vi "Create.vi"(8 "error in (no error)":errorcluster) -> (0 "error out":errorcluster, 3 "Mock Result Observer out":refnum<class "Mock Result Observer.lvclass">)   [LabVIEW 2020, in "Mock Result Observer.lvclass"]
uses:
  Mock Result Observer.lvclass
  Result/Result.ctl
  Result/Status.ctl
  Result/Type.ctl
  Mock Result Observer.lvclass/Mock Result Observer.ctl
  Result/Result.lvlib
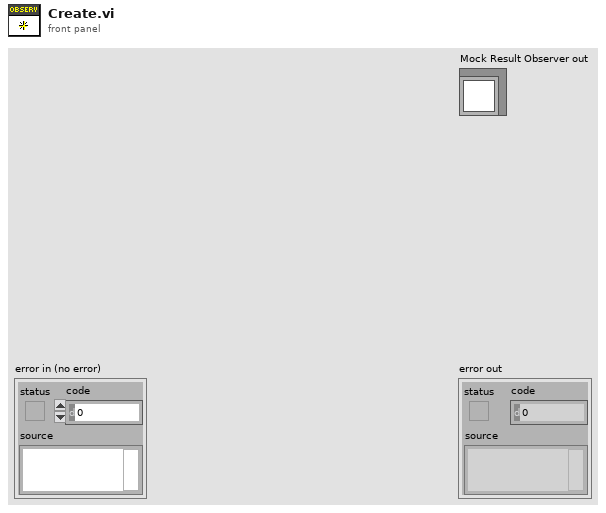
[diagram p1: front panel]
types:
  T1 = typedef "Result.lvlib/Result.ctl" = cluster{"Name":string, "Message":string, "Description":string, "Status":T2, "Result Type":T3, "Execution Time":dbl}
  T2 = typedef "Result.lvlib/Status.ctl" = enum16{"", "Passed", "Failed", "Error", "Skipped", "Setup Error", "Broken", "Teardown Error"}
  T3 = typedef "Result.lvlib/Type.ctl" = enum16{"Method", "Case", "Suite", "Pass", "Fail", "Skip", "Pass if", "Fail if", "Pass if Error", "Fail if Error", "Pass if Equal", "Fail if Equal"}
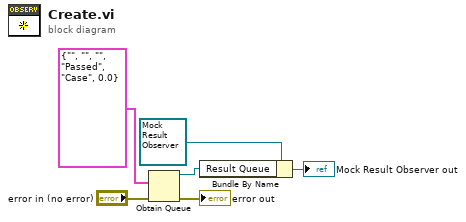
[diagram p0: block diagram]
diagram:
  n1 = Obtain Queue(element data type=T1 {"Name"="", "Message"="", "Description"="", "Status"=enum."Passed", "Result Type"=enum."Case", "Execution Time"=0.0} ("Result"), error in (no error)="error in (no error)") -> (queue out=w1:refnum<queue>, error out=→"error out":errorcluster)  [unwired: 3 in, 1 out]
  n2 = Bundle By Name(cluster=refnum<class "Mock Result Observer.lvclass"> refnum ("Mock Result Observer in"), "Result Queue"=w1) -> (→"Mock Result Observer out":refnum<class "Mock Result Observer.lvclass">)
